vi "Initialize.vi"(8 "error in (no error)":errorcluster, 11 "GA-Extend-Cmd in":refnum<class "GA-Extend-Cmd.lvclass">) -> (0 "error out":errorcluster, 3 "GA-Extend-Cmd out":refnum<class "GA-Extend-Cmd.lvclass">)   [LabVIEW 2013, in "GA-Extend-Cmd.lvclass"]
uses:
  GA-Extend-Cmd.lvclass
  States/GA-Extending-State/GrabberArms-ExtendingState.lvclass
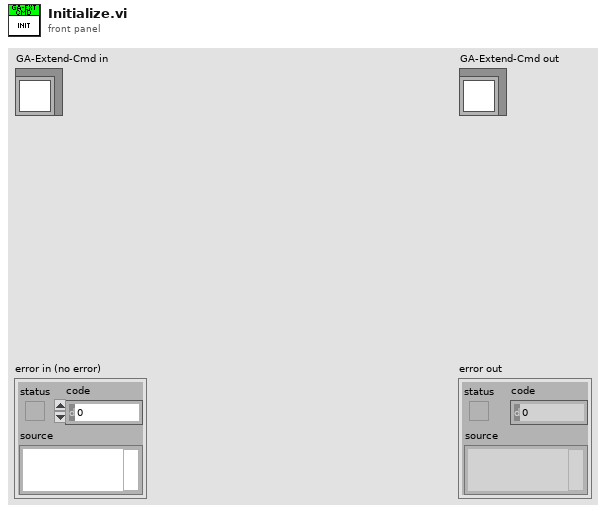
[diagram p1: front panel]
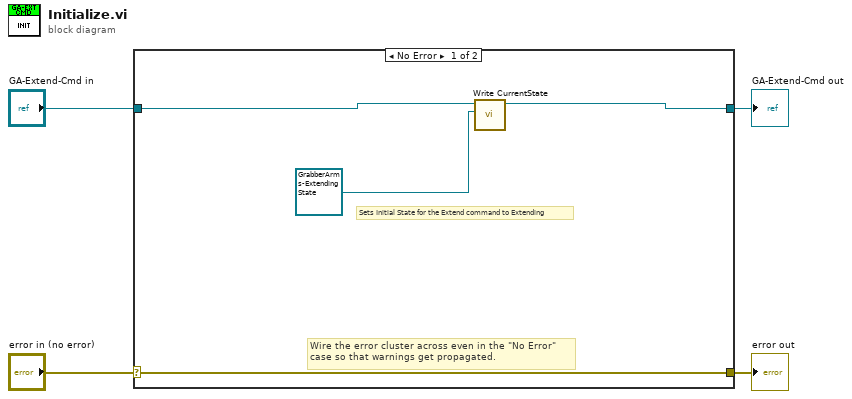
[diagram p0: block diagram]
diagram:
  n1 = case shown="No Error" "error in (no error)" {
    selector: "error in (no error)" -> [w8 w10]
    tunnel: [w8 w10] -> w3
    tunnel: [w6 w9] -> w1
    tunnel: "GA-Extend-Cmd in" -> [w7 w9]
    frame No Error {
      # "Sets Initial State for the Extend command to Extending"
      # "Wire the error cluster across even in the \"No Error\"\ncase so that warnings get propagated."
      n2 = call-dynamic "Write CurrentState.vi"("State.lvclass"=refnum<class "GrabberArms-ExtendingState.lvclass"> refnum ("GrabberArms-ExtendingState.lvclass"), "Command in"=w7) -> ("Command out"=w6:refnum<class "GA-Extend-Cmd.lvclass">)  [unwired: 8 in, 1 out]
    }
    frame Error {
    }
  }
  "error out" <- w3
  "GA-Extend-Cmd out" <- w1
